vi "Processing.vi"() -> ()   [LabVIEW 2013]
panel:
  in  "CORRECT CLASS":T1(radio)
  out "PREDICTED CLASS":T2(radio)
  in  "is this your \nfirst session?":bool
  in  "Choose your \nAlgorithm":u16(ring) items=["1. \"Inc Samples\" Algo.", "2.  \"Raw Spectrogram\" Algo.", "3. \"Elimination 1\" Algo.", "4. \"Elimination 2\" Algo."]
  in  "Cancel\n Retraining":bool
  out "correct class":dbl
  in  "stop":bool
  out "Predicted Class":dbl
  in  "address":string="localhost"
  out "Signal 1":dynamicdata(graph)
  out "Signal 3":dynamicdata(graph)
  out "Signal 4":dynamicdata(graph)
  out "Signal 2":dynamicdata(graph)
  # "no"
  # "yes"
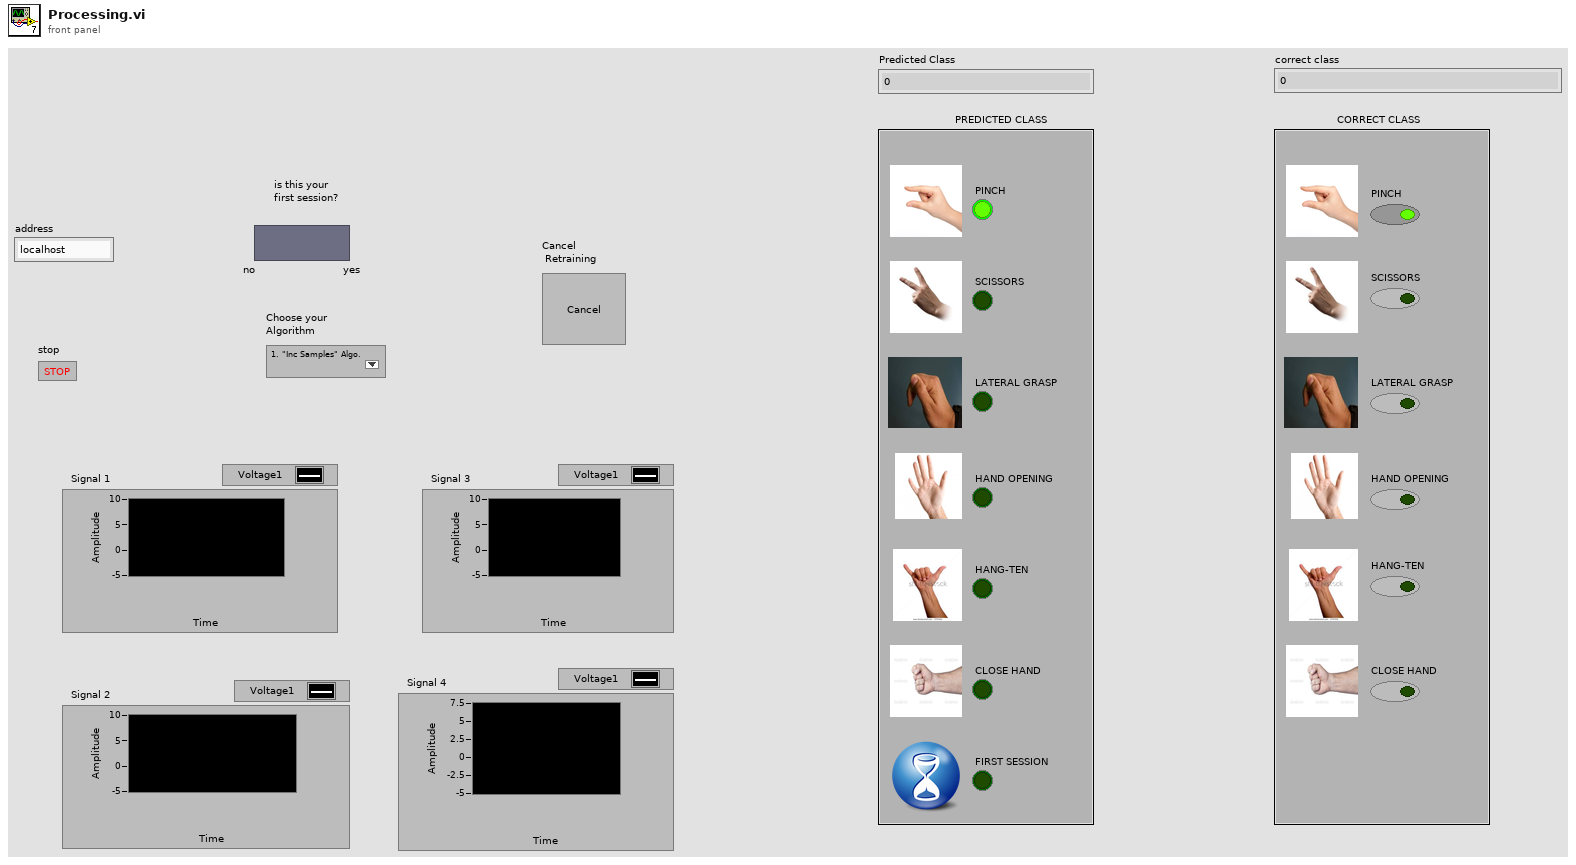
[diagram p1: front panel]
types:
  T1 = enum32{"PINCH", "SCISSORS", "LATERAL GRASP", "HAND OPENING", "HANG-TEN", "CLOSE HAND"}
  T2 = enum32{"PINCH", "SCISSORS", "LATERAL GRASP", "HAND OPENING", "HANG-TEN", "CLOSE HAND", "FIRST SESSION"}
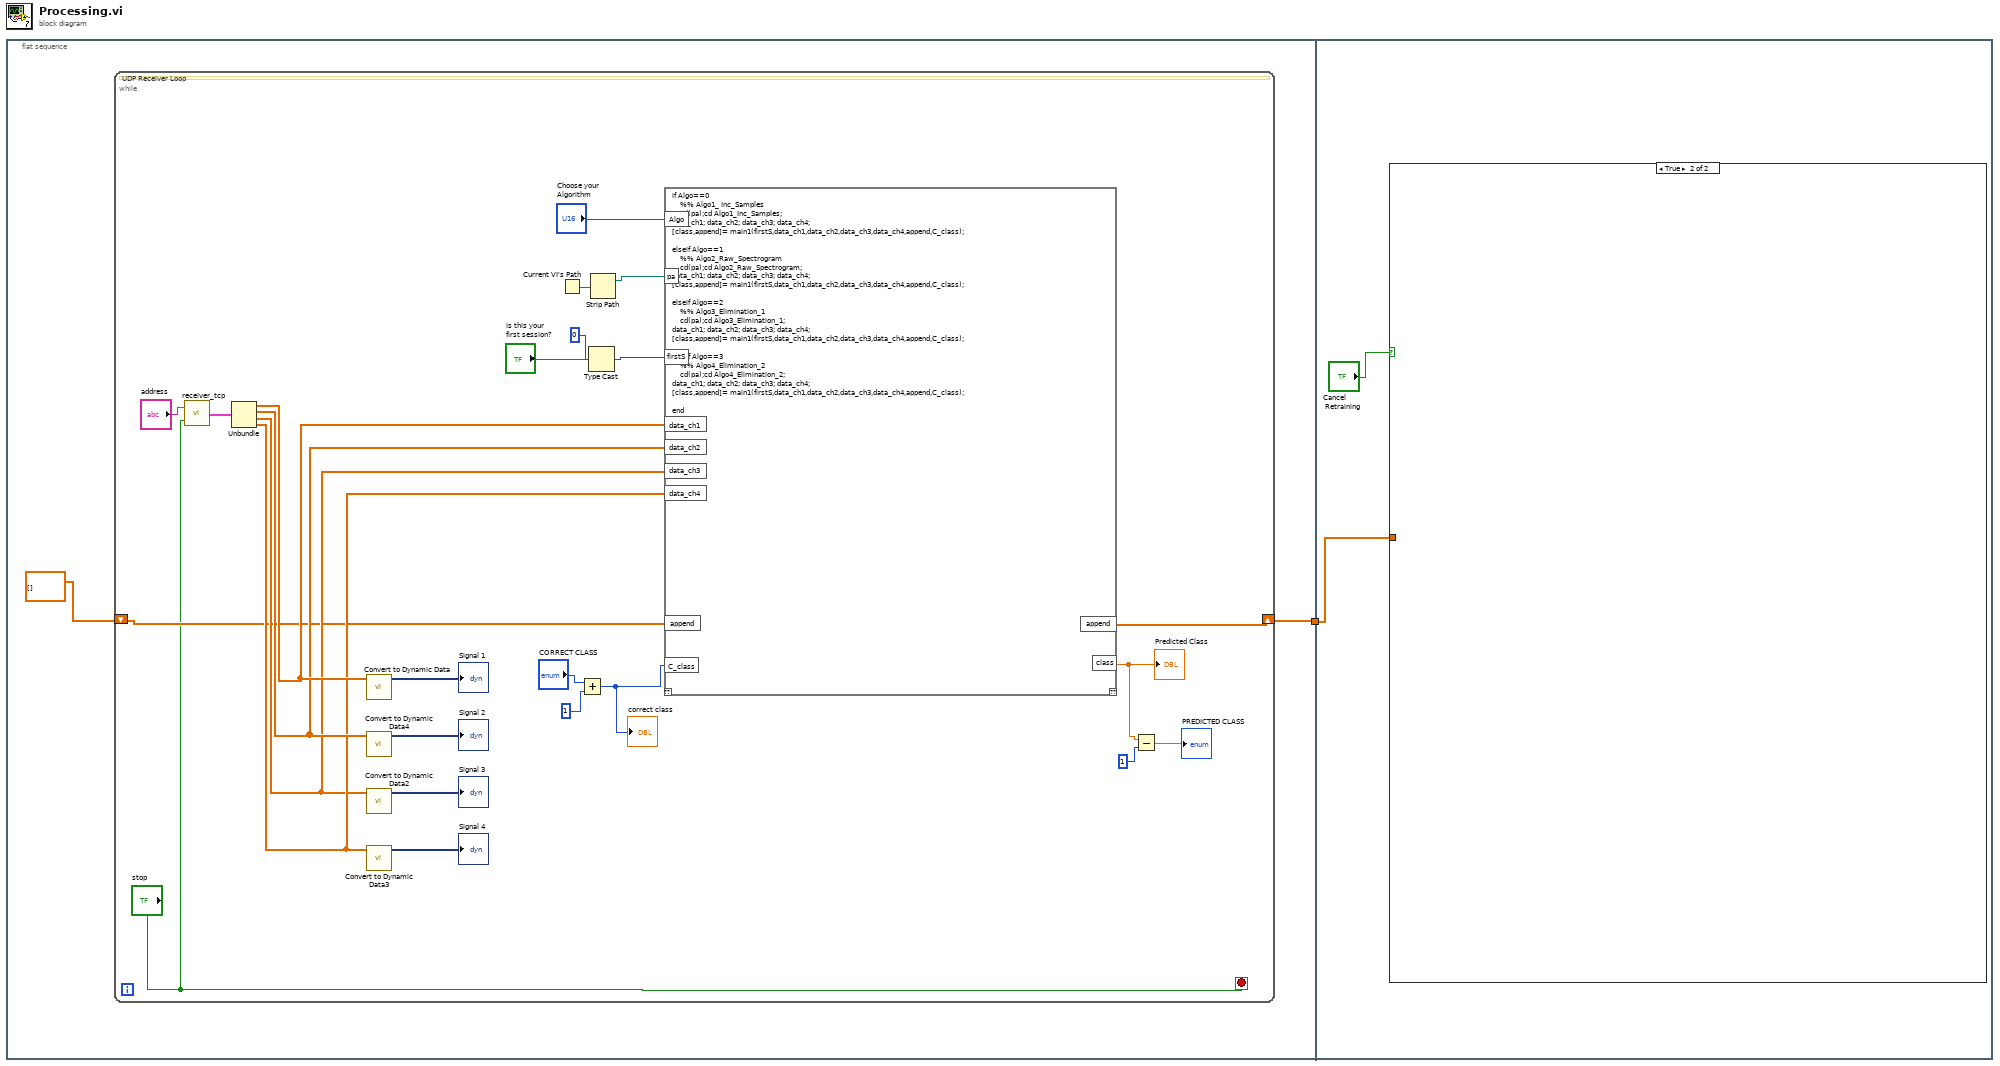
[diagram p0: block diagram]
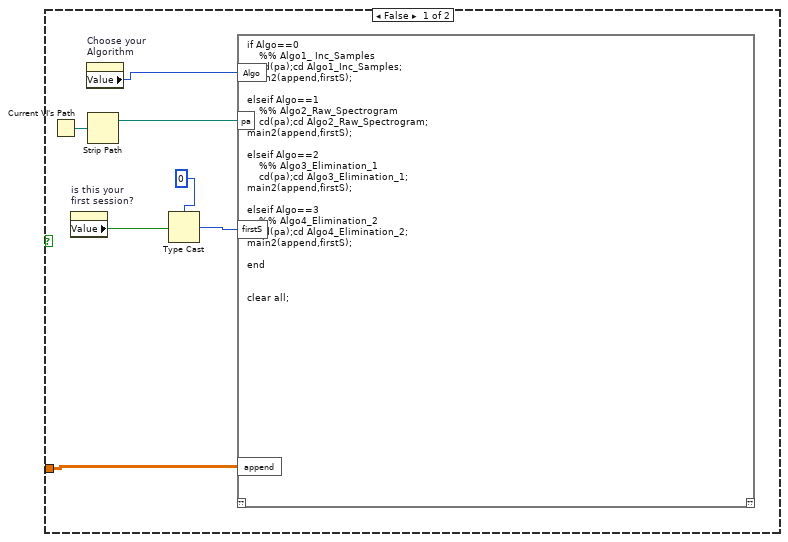
[diagram p2: hidden frame]
diagram:
  n1 = flat-sequence {
    tunnel: [w2] -> w1
    tunnel: w1 -> [w29]
    frame #0 {
      n2 = while {
        shift-right: [w17] -> w2
        shift-left: dbl[][] [] -> [w18]
        stop <- "stop" stop-if-true
        # "UDP Receiver Loop"
        n3 = call "receiver_tcp.vi"("stop"="stop", "String"="address") -> ("Cluster"=w16:cluster{dbl[], dbl[], dbl[], dbl[]})
        n4 = Unbundle(w16) -> (w22:dbl[], w21:dbl[], w19:dbl[], w20:dbl[])
        n5 = call "Convert to Dynamic Data"("Array"=w22) -> ("Dynamic Data Type"=→"Signal 1":dynamicdata)  [unwired: 3 in]
        n6 = call "Convert to Dynamic Data4"("Array"=w21) -> ("Dynamic Data Type"=→"Signal 2":dynamicdata)  [unwired: 3 in]
        n7 = call "Convert to Dynamic Data2"("Array"=w19) -> ("Dynamic Data Type"=→"Signal 3":dynamicdata)  [unwired: 3 in]
        n8 = call "Convert to Dynamic Data3"("Array"=w20) -> ("Dynamic Data Type"=→"Signal 4":dynamicdata)  [unwired: 3 in]
        n9 = Current VI's Path() -> (path=w28:path)
        n10 = Add(x="CORRECT CLASS", y=1) -> (x+y=w5:u32)
        "correct class" <- w5
        n11 = Type Cast(type=0, x="is this your \nfirst session?") -> (*(type *) &x=w12:i32)
        n12 = Strip Path(path=w28) -> (stripped path=w27:path)  [unwired: 1 out]
        n13 = script code="if Algo==0\n    %% Algo1_ Inc_Samples\n    cd(pa);cd Algo1_Inc_Samples;\ndata_ch1; data_ch2; data_ch3; data_ch4;\n[class,append]= main1(firstS,data_ch1,data_ch2,data_ch3,data_ch4,append,C_class);\n    \nelseif Algo==1\n    %% Algo2_Raw_Spectrogram\n    cd(pa);cd Algo2_Raw_Spectrogram;\ndata_ch1; data_ch2; data_ch3; data_ch4;\n[class,append]= main1(firstS,data_ch1,data_ch2,data_ch3,data_ch4,append,C_class);\n\nelseif Algo==2\n    %% Algo3_Elimination_1\n    cd(pa);cd Algo3_Elimination_1;\ndata_ch1; data_ch2; data_ch3; data_ch4;\n[class,append]= main1(firstS,data_ch1,data_ch2,data_ch3,data_ch4,append,C_class);\n\nelseif Algo==3\n    %% Algo4_Elimination_2\n    cd(pa);cd Algo4_Elimination_2;\ndata_ch1; data_ch2; data_ch3; data_ch4;\n[class,append]= main1(firstS,data_ch1,data_ch2,data_ch3,data_ch4,append,C_class);\n\nend"("data_ch1"=w22, "pa"=w27, "data_ch2"=w21, "data_ch3"=w19, "data_ch4"=w20, "append"=w18, "C_class"=w5, "firstS"=w12, "Algo"="Choose your \nAlgorithm") -> ("class"=w10:dbl, "append"=w17:dbl[][])  [unwired: 1 in, 1 out]
        "Predicted Class" <- w10
        n14 = Subtract(x=w10, y=1) -> (x-y=→"PREDICTED CLASS":dbl)
      }
    }
    frame #1 {
      n15 = case shown="True" "Cancel\n Retraining" {
        tunnel: w29 -> [w37 _]
        frame False {
          n16 = Current VI's Path() -> (path=w36:path)
          n17 = property on="is this your \nfirst session?" class="Bool (strict)"() -> ("Value"=w33:bool)  [unwired: 2 in, 2 out]
          n18 = property on="Choose your \nAlgorithm" class="Ring (strict)"() -> ("Value"=w31:u16)  [unwired: 2 in, 2 out]
          n19 = Strip Path(path=w36) -> (stripped path=w35:path)  [unwired: 1 out]
          n20 = Type Cast(type=0, x=w33) -> (*(type *) &x=w32:i32)
          n21 = script code="if Algo==0\n    %% Algo1_ Inc_Samples\n    cd(pa);cd Algo1_Inc_Samples;\nmain2(append,firstS);\n    \nelseif Algo==1\n    %% Algo2_Raw_Spectrogram\n    cd(pa);cd Algo2_Raw_Spectrogram;\nmain2(append,firstS);\n\nelseif Algo==2\n    %% Algo3_Elimination_1\n    cd(pa);cd Algo3_Elimination_1;\nmain2(append,firstS);\n\nelseif Algo==3\n    %% Algo4_Elimination_2\n    cd(pa);cd Algo4_Elimination_2;\nmain2(append,firstS);\n\nend\n   \n\nclear all;"("append"=w37, "pa"=w35, "firstS"=w32, "Algo"=w31) -> ()  [unwired: 1 in, 1 out]
        }
        frame True {
        }
      }
    }
  }
